vi "class_data.vi"() -> ()   [LabVIEW 2010, in "GenericDAQ.lvclass"]
uses:
  GenericDAQ.lvclass
panel:
  in  "latest instance":refnum<class "GenericDAQ.lvclass">
  in  "locked by":string
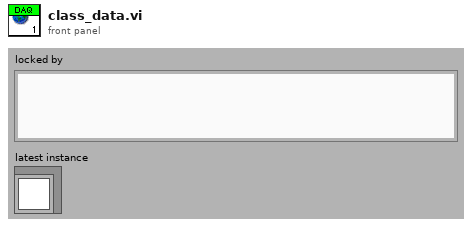
[diagram p1: front panel]
diagram:
